vi "SETREL_Status.vi"(0 "VisaCluster":T1, 11 "error in (no error)":errorcluster) -> (4 "VisaCluster":T1, 6 "Numeric":dbl, 8 "Answer":string, 15 "error out":errorcluster)   [LabVIEW 2014, in "FH 55.lvlib"]
uses:
  FH 55.lvlib
  TypeDef/VisaCluster.ctl
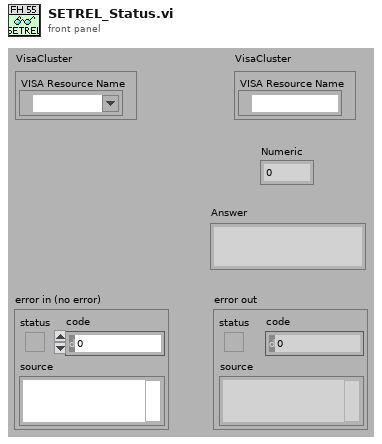
[diagram p1: front panel]
types:
  T1 = typedef "FH 55.lvlib/VisaCluster.ctl" = cluster{"VISA Resource Name":refnum<visa-resource-name>}
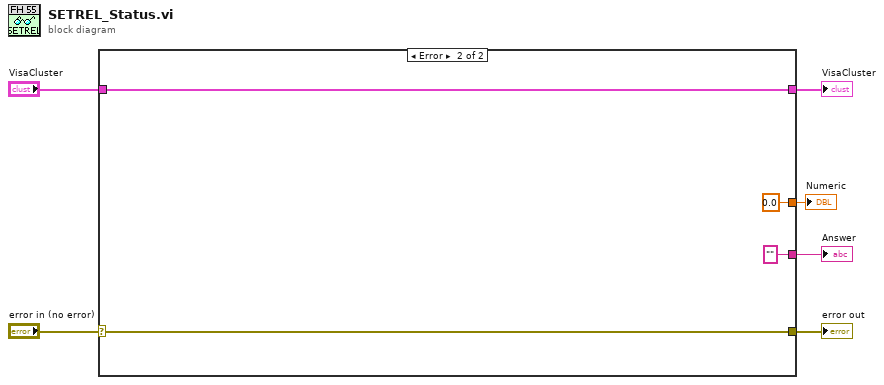
[diagram p0: block diagram]
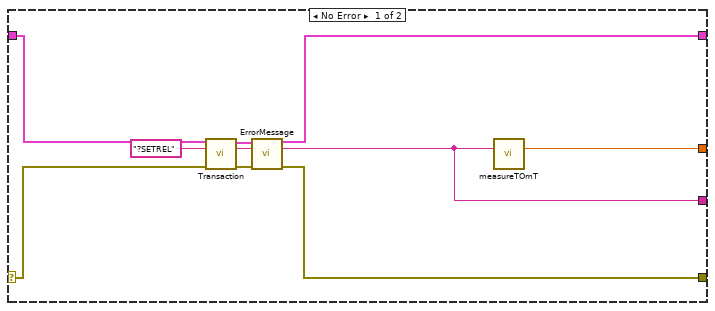
[diagram p2: hidden frame]
diagram:
  n1 = case shown="Error" "error in (no error)" {
    selector: "error in (no error)" -> [w9 w19]
    tunnel: "VisaCluster" -> [w10 w20]
    tunnel: [w16 w20] -> w2
    tunnel: [w11 w19] -> w4
    tunnel: [w7 ""] -> w3
    tunnel: [w8 0.0 ("Numeric")] -> w1
    frame No Error {
      n2 = call "Transaction.vi"("VisaCluster"=w10, "Command"="?SETREL", "error in (no error)"=w9) -> ("VisaCluster"=w14:T1, "Answer"=w12:string, "error out"=w15:errorcluster)  [unwired: 9 in, 1 out]
      n3 = call "ErrorMessage.vi"("VisaCluster"=w14, "Message In"=w12, "error in (no error)"=w15) -> ("VisaCluster"=w16:T1, "Message Out"=w7:string, "error out"=w11:errorcluster)  [unwired: 10 in]
      n4 = call "measureTOmT.vi"("string"=w7) -> ("Numeric"=w8:dbl)  [unwired: 12 in, 2 out]
    }
    frame Error {
    }
  }
  "error out" <- w4
  "Answer" <- w3
  "VisaCluster" <- w2
  "Numeric" <- w1
